vi "compute_slopes_from_image.vi"() -> ()   [LabVIEW 2018]
uses:
  <userlib>/WaveKit.lib/Classes/HasoEngine/HasoEngine.lvclass
  <userlib>/WaveKit.lib/Classes/Image/Image.lvclass
  <userlib>/WaveKit.lib/Controls/SlopesEngineSetup.ctl
  <userlib>/WaveKit.lib/Controls/Point2D.ctl
  <userlib>/WaveKit.lib/Controls/HasoSlopes.lvclass
panel:
  in  "Output folder":path=path "D:/Data/20200122_Test"
  in  "Camera image file":path=path "C:/Program Files (x86)/Imagine Optic/WaveKit/Labview/Examples/Data/data_image.himg"
  in  "Haso configuration file":path=path "C:/Program Files (x86)/Imagine Optic/WaveKit/Labview/Examples/Data/config_file_haso.dat"
  out "Y Slopes":sgl[][](graph)
  in  "Output file name":string="test.has"
  out "X Slopes":sgl[][](graph)
  out "error out":errorcluster
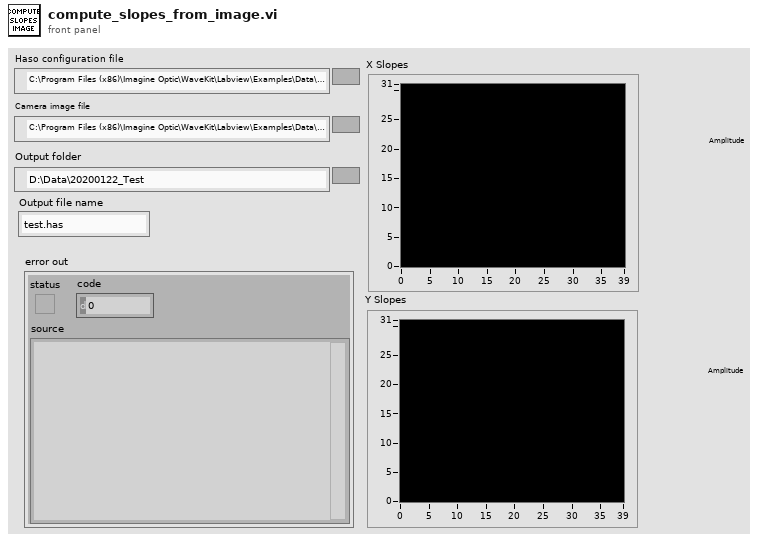
[diagram p1: front panel]
types:
  T1 = typedef "SlopesEngineSetup.ctl" = cluster{"Start sub-aperture":T2, "Pupil average":dbl}
  T2 = typedef "Point2D.ctl" = cluster{"X":u32, "Y":u32}
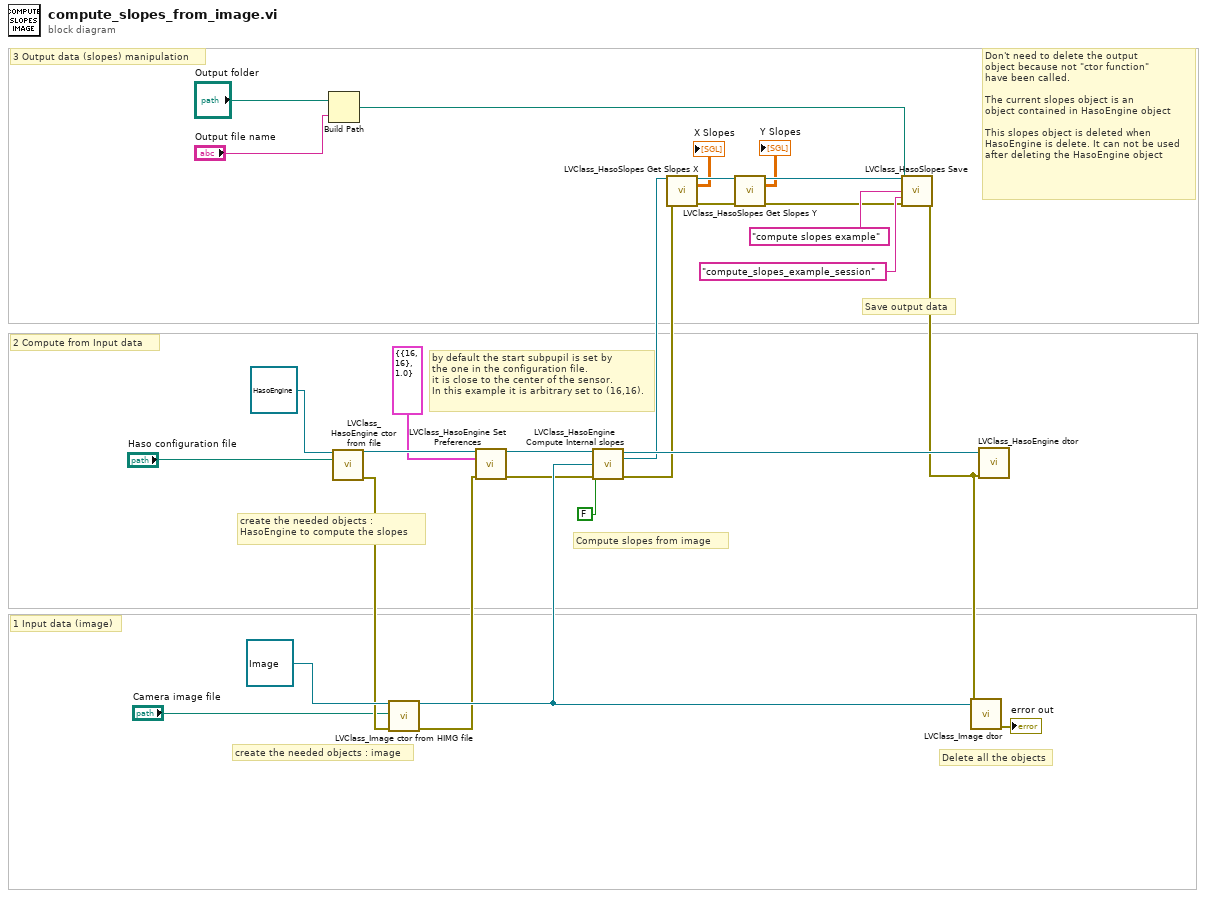
[diagram p0: block diagram]
diagram:
  # "Don't need to delete the output\nobject because not \"ctor function\"\nhave been called.\n\nThe current slopes object is an \nobject contained in HasoEngine object\n\nThis slopes object is deleted when \nHasoEngine is delete. It can not be used\nafter deleting the HasoEngine object"
  # "Save output data"
  # "create the needed objects : \nHasoEngine to compute the slopes"
  # "3 Output data (slopes) manipulation"
  # "2 Compute from Input data"
  # "1 Input data (image)"
  # "Delete all the objects"
  # "Compute slopes from image"
  # "by default the start subpupil is set by \nthe one in the configuration file. \nit is close to the center of the sensor.\nIn this example it is arbitrary set to (16,16)."
  # "create the needed objects : image"
  n1 = Build Path(base path="Output folder", name or relative path="Output file name") -> (appended path=w3:path)
  n2 = call <userlib>:"LVClass_HasoEngine ctor from file.vi"("HasoEngine in"=refnum<class "HasoEngine.lvclass"> refnum, "Configuration file path"="Haso configuration file") -> ("HasoEngine out"=w26:refnum<class "HasoEngine.lvclass">, "error out"=w17:errorcluster)  [unwired: 12 in]
  n3 = call <userlib>:"LVClass_Image ctor from HIMG file.vi"("Image in"=refnum<class "Image.lvclass"> refnum, "Path to image file"="Camera image file", "error in (no error)"=w17) -> ("Image out"=w18:refnum<class "Image.lvclass">, "error out"=w16:errorcluster)  [unwired: 11 in]
  n4 = call <userlib>:"LVClass_HasoEngine Set Preferences.vi"("HasoEngine in"=w26, "Slopes_HasoEngine_Setup"=T1 {"Start sub-aperture"={"X"=16, "Y"=16}, "Pupil average"=1.0}, "error in (no error)"=w16) -> ("HasoEngine out"=w24:refnum<class "HasoEngine.lvclass">, "error out"=w15:errorcluster)  [unwired: 11 in]
  n5 = call <userlib>:"LVClass_HasoEngine Compute Internal slopes.vi"("HasoEngine in"=w24, "Image.lvclass"=w18, "learn_from_trimmer"=FALSE, "error in (no error)"=w15) -> ("HasoEngine out"=w20:refnum<class "HasoEngine.lvclass">, "HasoSlopes (dup)"=w11:refnum<class "HasoSlopes.lvclass">, "error out"=w7:errorcluster)  [unwired: 7 in, 2 out]
  n6 = call <userlib>:"LVClass_HasoSlopes Get Slopes X.vi"("HasoSlopes in"=w11, "error in (no error)"=w7) -> ("HasoSlopes out"=w13:refnum<class "HasoSlopes.lvclass">, "Slopesx"=→"X Slopes":sgl[][], "error out"=w12:errorcluster)  [unwired: 11 in]
  n7 = call <userlib>:"LVClass_HasoSlopes Get Slopes Y.vi"("HasoSlopes in"=w13, "error in (no error)"=w12) -> ("HasoSlopes out"=w10:refnum<class "HasoSlopes.lvclass">, "Slopesy"=→"Y Slopes":sgl[][], "error out"=w6:errorcluster)  [unwired: 11 in]
  n8 = call <userlib>:"LVClass_HasoSlopes Save.vi"("HasoSlopes in"=w10, "path"=w3, "comments"="compute slopes example", "session"="compute_slopes_example_session", "error in (no error)"=w6) -> ("error out"=w19:errorcluster)  [unwired: 9 in, 1 out]
  n9 = call <userlib>:"LVClass_Image dtor.vi"("Image in"=w18, "error in (no error)"=w19) -> ("error out"=→"error out":errorcluster)  [unwired: 12 in, 1 out]
  n10 = call <userlib>:"LVClass_HasoEngine dtor.vi"("HasoEngine in"=w20, "error in (no error)"=w19) -> ()  [unwired: 12 in, 2 out]
